vi "SMTP Notification.vi"() -> ()   [LabVIEW 2017]
uses:
  <vilib>/smtpClient/Set Message Text.vi
  <vilib>/smtpClient/LabVIEWSMTPClient.lvlib
panel:
  in  "plain text message":string
  in  "subject":string
  in  "To":string
  in  "use TLS (false)":bool
  in  "password":string
  in  "username":string
  in  "from":string
  in  "Port":string
  in  "Outgoing mail SMTP":string
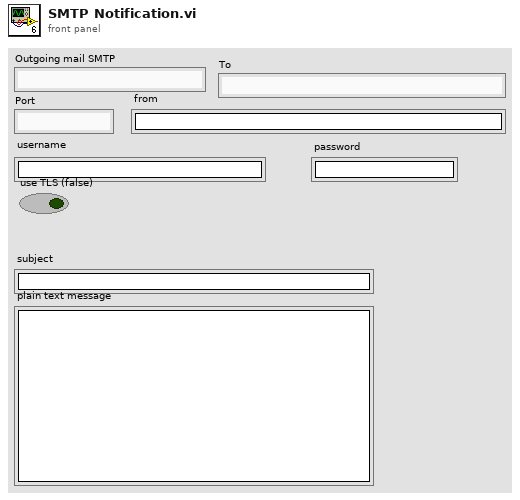
[diagram p1: front panel]
types:
  T1 = typedef "LabVIEWSMTPClient.lvlib/SmtpClientHandle.ctl" = refnum<k1>
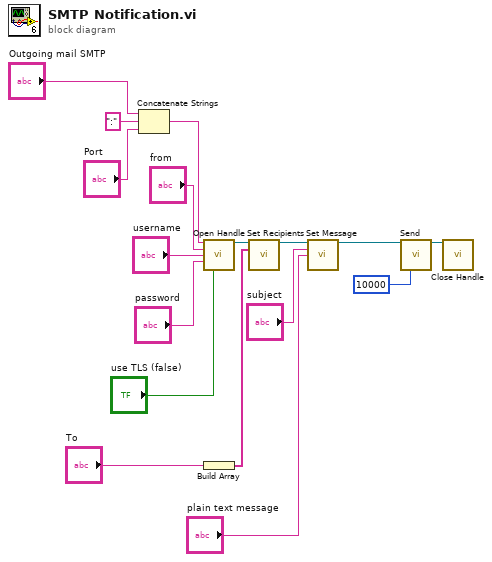
[diagram p0: block diagram]
diagram:
  n1 = Concatenate Strings("Outgoing mail SMTP", ":" ("string"), "Port") -> (w10:string)
  n2 = call <vilib>:"Open Handle.vi"("server address"=w10, "from"="from", "username"="username", "password"="password", "use TLS (false)"="use TLS (false)") -> ("handle out"=w17:T1)  [unwired: 9 in, 1 out]
  n3 = Build Array("To") -> (w5:string[])
  n4 = call <vilib>:"Set Recipients.vi"("handle in"=w17, "to"=w5) -> ("handle out"=w16:T1)  [unwired: 12 in, 1 out]
  n5 = call-poly <vilib>:"Set Message.vi"("handle in"=w16, "subject"="subject", "plain text message"="plain text message") -> ("handle out"=w15:T1)  [unwired: 11 in, 1 out]
  n6 = call <vilib>:"Send.vi"("handle in"=w15, "timeout in ms (10000)"=10000) -> ("handle out"=w14:T1)  [unwired: 11 in, 2 out]
  n7 = call <vilib>:"Close Handle.vi"("handle in"=w14) -> ()  [unwired: 13 in, 2 out]
